vi "ARP1762.vi"() -> ()   [LabVIEW 2012]
uses:
  <vilib>/Utility/file.llb/Write To Spreadsheet File (DBL).vi
panel:
  in  "AP Sweep Width (MHz)":dbl
  in  "Time (ms)":dbl
  in  "Recooling Time":u32
  out "binned path":path=path "c:/data/1762 Scans/2016-08-24-scans/2016-08-24_15-56-18_1762scanWithPumping.txt"
  out "Path":path=path "c:/data/1762 Scans/2016-08-24_15-56-18_1762scanWithPumping.txt"
  in  "PMT Sample Time (secs)":dbl=0.05 format="%0.2f"
  in  "Stop Scan":bool
  in  "Delete Data":bool
  out "ExptWvfm":digitalwaveform(waveform)={"t0"=timestamp(0 s since 1904-01-01), "dt"=1e-07, "Y"={"transitions"=[0, 2100, 2200, 2300, 2301, 2311, 2361, 2461], "data"=[[1, 1, 1, 0, 0], [1, 0, 1, 0, 0], [1, 0, 0, 0, 0], [0, 0, 0, 0, 0], [0, 0, 0, 0, 0], [0, 0, 0, 0, 1], [0, 0, 0, 0, 0], [0, 1, 1, 0, 0]]}, "error"={"status"=FALSE, "code"=37421928, "source"=""}}
  out "PMT Counts":i32(graph)=1168
  out "Counts after 1762":i32=1168
  out "OuterLoop":i32=40
  out "InnerLoop":i32=1
  in  "Freq Step Size (MHz)":dbl=0.02
  out "Bright Events":dbl
  in  "Discriminator Level\n (Bright/Dark)":i32=100
  out "digital waveform out 2":digitalwaveform(waveform)={"t0"=timestamp(0 s since 1904-01-01), "dt"=1e-07, "Y"={"transitions"=[0, 2100, 2200, 2300, 2301, 2311, 2361, 2461], "data"=[[1, 1, 1, 0, 0], [1, 0, 1, 0, 0], [1, 0, 0, 0, 0], [0, 0, 0, 0, 0], [0, 0, 0, 0, 0], [0, 0, 0, 0, 1], [0, 0, 0, 0, 0], [0, 1, 1, 0, 0]]}, "error"={"status"=FALSE, "code"=37421928, "source"=""}}
  in  "1762 pulse length\n (microsecs)":dbl=100.0
  in  "Comment":string=" "
  in  "B Field":dbl=999.0
  in  "RF Power":dbl=999.0
  in  "Runs per data point":dbl=15.0
  in  "Low Freq (MHz)":dbl(slide)=80.0 min=80.0 max=90.0 step=5e-05 scale=80.0..90.0 scale format="%#.5f"
  in  "High Freq (MHz)":dbl(slide)=90.0 min=77.0 max=93.0 step=5e-05 scale=80.0..90.0 scale format="%#.0f"
  out "Cur Freq":dbl=84890000.0 format="%#_8f"
  out "Frequency Scan":cluster{dbl, dbl}[](graph)=[{85300000.0, 1.0}, {85290000.0, 1.0}, {85280000.0, 1.0}, {85270000.0, 1.0}, {85260000.0, 1.0}, {85250000.0, 1.0}, {85240000.0, 1.0}, {85230000.0, 1.0}, {85220000.0, 1.0}, {85210000.0, 1.0}, {85200000.0, 1.0}, {85190000.0, 1.0}, {85180000.0, 1.0}, {85170000.0, 1.0}, {85160000.0, 1.0}, {85150000.0, 1.0}, {85140000.0, 1.0}, {85130000.0, 1.0}, {85120000.0, 1.0}, {85110000.0, 1.0}, {85100000.0, 1.0}, {85090000.0, 1.0}, {85080000.0, 1.0}, {85070000.0, 1.0}, {85060000.0, 1.0}, {85050000.0, 1.0}, {85040000.0, 1.0}, {85030000.0, 1.0}, {85020000.0, 1.0}, {85010000.0, 1.0}, {85000000.0, 1.0}, {84990000.0, 1.0}, {84980000.0, 1.0}, {84970000.0, 1.0}, {84960000.0, 1.0}, {84950000.0, 1.0}, {84940000.0, 1.0}, {84930000.0, 1.0}, {84920000.0, 1.0}, {84910000.0, 1.0}, {84900000.0, 1.0}]
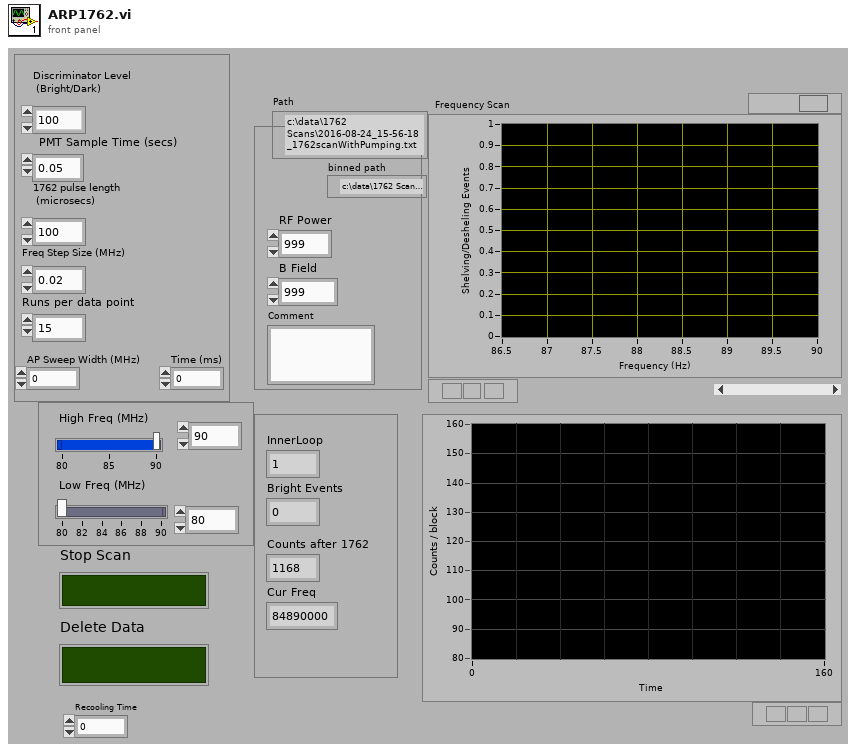
[diagram p1: front panel]
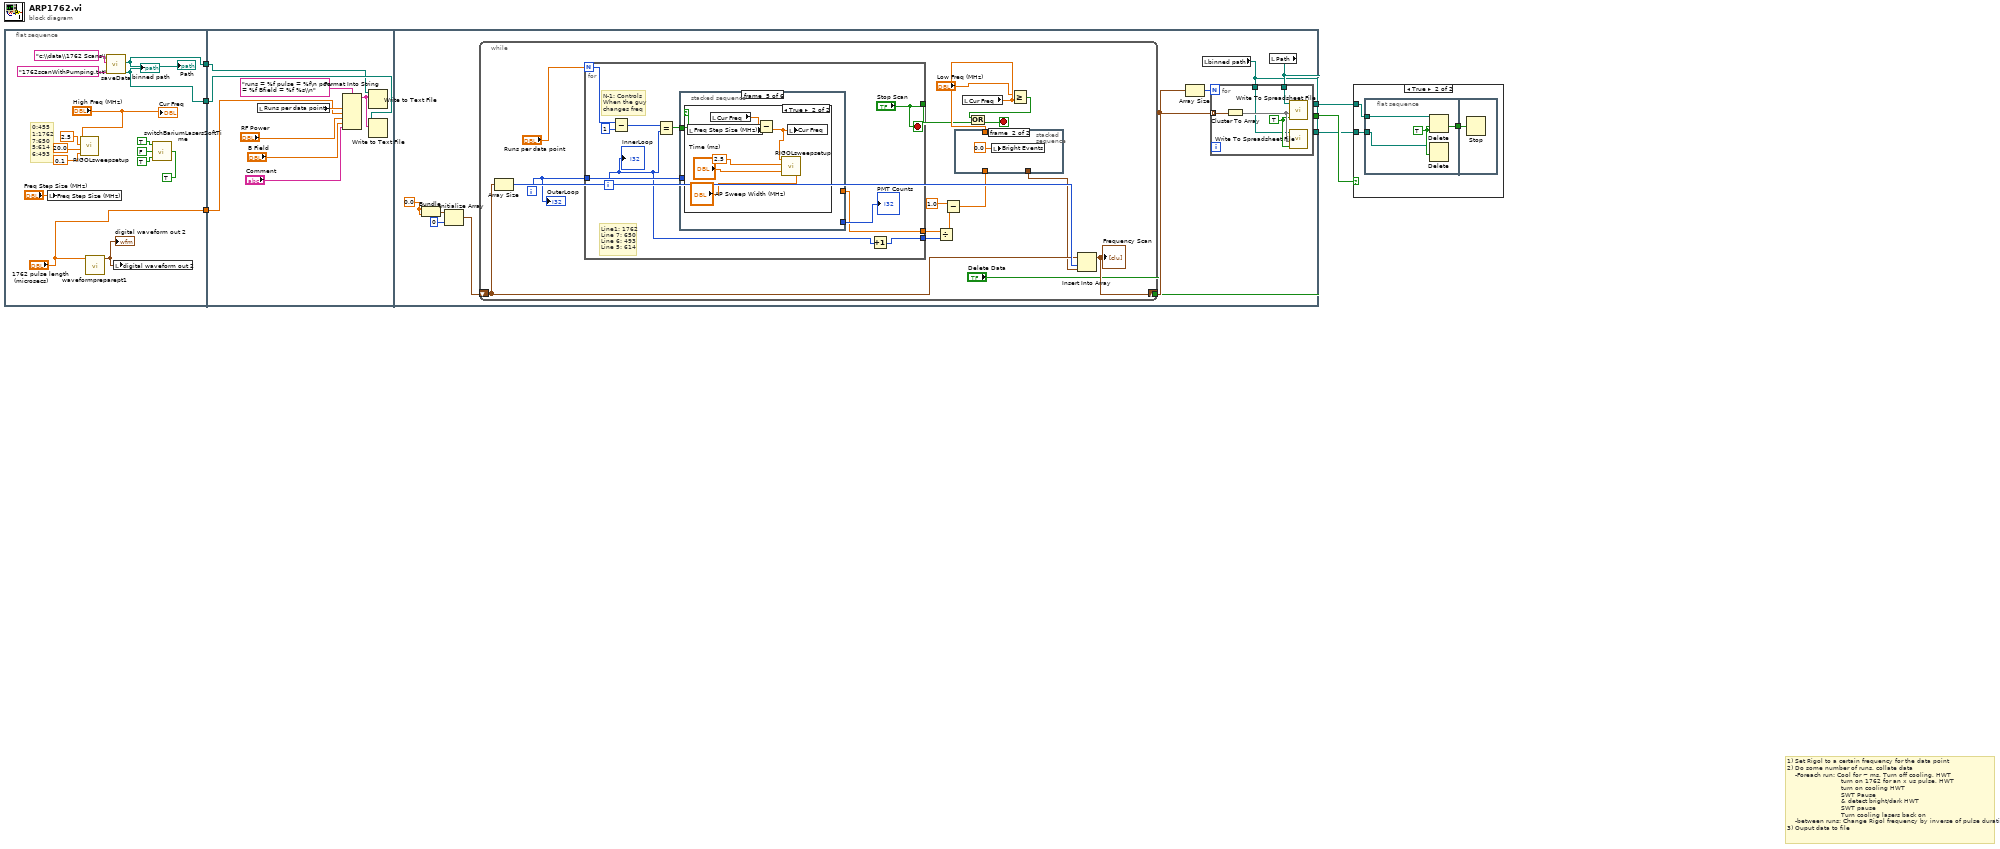
[diagram p0: block diagram]
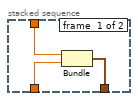
[diagram p3: hidden frame]
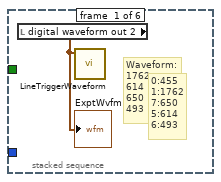
[diagram p4: hidden frame]
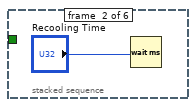
[diagram p5: hidden frame]
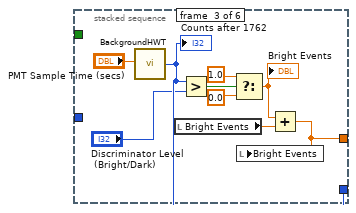
[diagram p6: hidden frame]
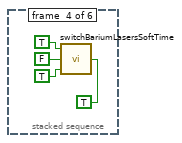
[diagram p7: hidden frame]
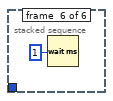
[diagram p9: hidden frame]
diagram:
  # "1) Set Rigol to a certain frequency for the data point\n2) Do some number of runs, collate data\n    -Foreach run: Cool for ~ ms, Turn off cooling, HWT\n                           turn on 1762 for an x us pulse, HWT\n                           turn on cooling HWT\n                           SWT Pause\n                           & detect bright/dark HWT\n                           SWT pause\n                           Turn cooling lasers back on \n    -between runs: Change Rigol frequency by inverse of pulse duration\n3) Ouput data to file"
  n1 = flat-sequence {
    tunnel: [w18] -> w6
    tunnel: ["1762 pulse length\n (microsecs)"] -> w5
    tunnel: [w15] -> w4
    tunnel: w6 -> [w30]
    tunnel: w5 -> [w24]
    tunnel: w4 -> [w22]
    tunnel: [w33] -> w3
    tunnel: [w32] -> w2
    tunnel: [w31] -> w1
    frame #0 {
      # "0:455\n1:1762\n7:650\n5:614\n6:493"
      n2 = local write "Freq Step Size (MHz)"("Freq Step Size (MHz)") -> ()
      n3 = call "RIGOLsweepsetup.vi"("AP Sweep Width (MHz)"=0.1, "Time (ms)"=20.0, "Amplitude (Vpp)"=2.5, "Frequency (MHz)"="High Freq (MHz)") -> ()  [unwired: 8 in]
      n4 = call "waveformpreparept1.vi"("1762 pulse length (units of 1 us)"="1762 pulse length\n (microsecs)") -> ("digital waveform out 2"=w20:digitalwaveform)  [unwired: 8 in]
      "digital waveform out 2" <- w20
      n5 = call "saveData.vi"("filename"="1762scanWithPumping.txt", "dataDirectory"="c:\\data\\1762 Scans\\") -> ("binned path"=w18:path, "Path"=w15:path)  [unwired: 8 in]
      "Path" <- w15
      "binned path" <- w18
      n6 = local write "digital waveform out 2"(w20) -> ()
      n7 = call "switchBariumLasersSoftTime.vi"("650"=TRUE, "614"=TRUE, "1762"=FALSE, "493"=TRUE) -> ()  [unwired: 2 in]
      "Cur Freq" <- "High Freq (MHz)"
    }
    frame #1 {
      n8 = local read "Runs per data point"() -> (w28:dbl)
      n9 = Format Into String(format string="runs = %f pulse = %f\n pow = %f Bfield = %f %s\\n", w28, w24, "RF Power", "B Field", "Comment") -> (resulting string=w23:string)  [unwired: 2 in, 1 out]
      n10 = Write to Text File(file (use dialog)=w22, text=w23) -> ()  [unwired: 2 in, 3 out]
      n11 = Write to Text File(file (use dialog)=w30, text=w23) -> ()  [unwired: 2 in, 3 out]
    }
    frame #2 {
      w38 = 0.0
      n12 = Bundle(w38, w38) -> (w39:cluster{dbl, dbl})  [unwired: 1 in]
      n13 = Initialize Array(w39, 0) -> (w36:cluster{dbl, dbl}[])
      n14 = while {
        shift-right: [w59] -> w34
        shift-left: w36 -> [w60]
        tunnel: ["Delete Data"] -> w33
        i -> [w58]
        stop <- w51 stop-if-true
        n15 = Array Size(array=w60) -> (size(s)=w61:i32)
        n16 = for {
          N: "Runs per data point" -> [w72]
          tunnel: [w69] -> w55
          tunnel: w58 -> [w68]
          tunnel: ["Stop Scan"] -> w53
          tunnel: [w66] -> w45
          i -> [w67]
          stop <- "Stop Scan" stop-if-true
          # "Line1: 1762\nLine 7: 650\nLine 6: 493\nLine 5: 614"
          # "N-1: Controls\nWhen the guy\nchanges freq"
          n17 = Subtract(x=w72, y=1) -> (x-y=w75:i32)
          n18 = Equal?(x=w75, y=w67) -> (x = y?=w73:bool)
          n19 = stacked-sequence {
            tunnel: w68 -> [_ _ _ _ _ _]
            tunnel: [_ _ w82 _ _ _] -> w71
            tunnel: w73 -> [_ _ _ _ w91 _]
            tunnel: [_ _ w78 _ _ _] -> w69
            frame #0 {
              # "0:455\n1:1762\n7:650\n5:614\n6:493"
              # "Waveform:\n1762\n614\n650\n493"
              n20 = local read "digital waveform out 2"() -> (w76:digitalwaveform)
              "ExptWvfm" <- w76
              n21 = call "LineTriggerWaveform.vi"("digital waveform in"=w76) -> ()  [unwired: 11 in]
            }
            frame #1 {
              n22 = Wait (ms)(milliseconds to wait="Recooling Time") -> ()  [unwired: 1 out]
            }
            frame #2 {
              n23 = call "BackgroundHWT.vi"("Sample Time(seconds)"="PMT Sample Time (secs)") -> ("Counts"=w82:i32)
              "Counts after 1762" <- w82
              n24 = local read "Bright Events"() -> (w83:dbl)
              n25 = Greater?(x=w82, y="Discriminator Level\n (Bright/Dark)") -> (0:w80:bool)
              n26 = Select(t=1.0, s=w80, f=0.0) -> (s? t:f=w84:dbl)
              "Bright Events" <- w84
              n27 = Add(x=w84, y=w83) -> (x+y=w78:dbl)
              n28 = local write "Bright Events"(w78) -> ()
            }
            frame #3 {
              n29 = call "switchBariumLasersSoftTime.vi"("650"=TRUE, "614"=TRUE, "1762"=FALSE, "493"=TRUE) -> ()  [unwired: 2 in]
            }
            frame #4 {
              n30 = case shown="True" w91 {
                frame False {
                }
                frame True {
                  n31 = local read "Freq Step Size (MHz)"() -> (w96:dbl)
                  n32 = local read "Cur Freq"() -> (w97:dbl)
                  n33 = Subtract(x=w97, y=w96) -> (x-y=w94:dbl)
                  n34 = call "RIGOLsweepsetup.vi"("AP Sweep Width (MHz)"="AP Sweep Width (MHz)", "Time (ms)"="Time (ms)", "Amplitude (Vpp)"=2.5, "Frequency (MHz)"=w94) -> ()  [unwired: 8 in]
                  n35 = local write "Cur Freq"(w94) -> ()
                }
              }
            }
            frame #5 {
              n36 = Wait (ms)(milliseconds to wait=u32 1) -> ()  [unwired: 1 out]
            }
          }
          "PMT Counts" <- w71
          n37 = Increment(x=w67) -> (x+1=w66:i32)
          "InnerLoop" <- w67
        }
        n38 = Divide(x=w55, y=w45) -> (x/y=w47:dbl)
        n39 = Subtract(x=1.0, y=w47) -> (x-y=w46:dbl)
        n40 = local read "Cur Freq"() -> (w56:dbl)
        n41 = stacked-sequence {
          tunnel: w46 -> [w64 _]
          tunnel: [w63 _] -> w57
          tunnel: w56 -> [w62 _]
          frame #0 {
            n42 = Bundle("Cur Freq"=w62, w64) -> (w63:cluster{"Cur Freq":dbl, dbl})  [unwired: 1 in]
          }
          frame #1 {
            n43 = local write "Bright Events"(0.0 ("Bright Events")) -> ()
          }
        }
        n44 = Greater Or Equal?(x="Low Freq (MHz)", y=w56) -> (x >= y?=w50:bool)
        n45 = Or(x=w50, y=w53) -> (x .or. y?=w51:bool)
        n46 = Insert Into Array(array=w60, index=w61, new element=w57) -> (w59:cluster{dbl, dbl}[])
        "Frequency Scan" <- w59
        "OuterLoop" <- w58
      }
      n47 = Array Size(array=w34) -> (size(s)=w35:i32)
      n48 = local read "binned path"() -> (w31:path)
      n49 = local read "Path"() -> (w32:path)
      n50 = for {
        N: w35 -> [_]
        tunnel: w34 -> [w44] mode=indexing
        tunnel: w31 -> [w41]
        tunnel: w32 -> [w40]
        w42 = TRUE
        n51 = Cluster To Array(cluster=w44) -> (array=w43:dbl[])
        n52 = call-poly <vilib>:"Write To Spreadsheet File.vi"("append to file? (new file:F)"=w42, "1D data"=w43, "file path (dialog if empty)"=w40) -> ()  [unwired: 5 in, 1 out]
        n53 = call-poly <vilib>:"Write To Spreadsheet File.vi"("append to file? (new file:F)"=w42, "1D data"=w43, "file path (dialog if empty)"=w41) -> ()  [unwired: 5 in, 1 out]
      }
    }
  }
  n54 = case shown="True" w3 {
    tunnel: w2 -> [_ w100]
    tunnel: w1 -> [_ w99]
    frame False {
    }
    frame True {
      n55 = flat-sequence {
        tunnel: [w105] -> w101
        tunnel: w100 -> [w103]
        tunnel: w99 -> [w102]
        tunnel: w101 -> [w106]
        frame #0 {
          w104 = TRUE ("confirm (F)")
          n56 = Delete(path (use dialog)=w103, confirm (F)=w104) -> (cancelled=w105:bool)  [unwired: 3 in, 2 out]
          n57 = Delete(path (use dialog)=w102, confirm (F)=w104) -> ()  [unwired: 3 in, 3 out]
        }
        frame #1 {
          n58 = Stop(stop? (T)=w106) -> ()
        }
      }
    }
  }
